vi "HexStringToBoolArray.vi"(0 "Input String":string="FF 55 01", 5 "Fixed Output Size (bytes)":i32=-1, 7 "Reverse Endian?":bool, 11 "Error In":errorcluster) -> (4 "Output Array":bool[][](array[boolean])=[[TRUE, FALSE, FALSE, FALSE, FALSE, FALSE, FALSE, FALSE], [TRUE, FALSE, TRUE, FALSE, TRUE, FALSE, TRUE, FALSE], [TRUE, TRUE, TRUE, TRUE, TRUE, TRUE, TRUE, TRUE]], 15 "Error Out":errorcluster)   [LabVIEW 2016]
panel:
  out "u32 verified":u32=16733441 format="%08x"
  # "Set 'Reverse' if working with hex data where MSB is at end of string."
  # "Pads leading zeroes to output \na larger size, or trims MSB(s) to \noutput a smaller size.\nEx:  For Input \"FF 55 01\": \n       Size 3 yields 0xFF5501\n       Size 2 yields (u16) 0x5501\n       Size 4 yields (u32) 0x00FF5501\n\nDefault (-1) maintains the input size"
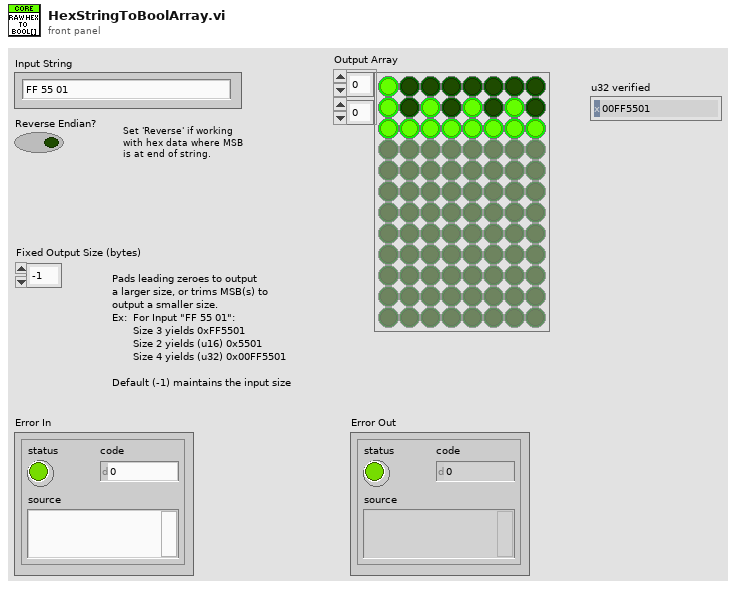
[diagram p1: front panel]
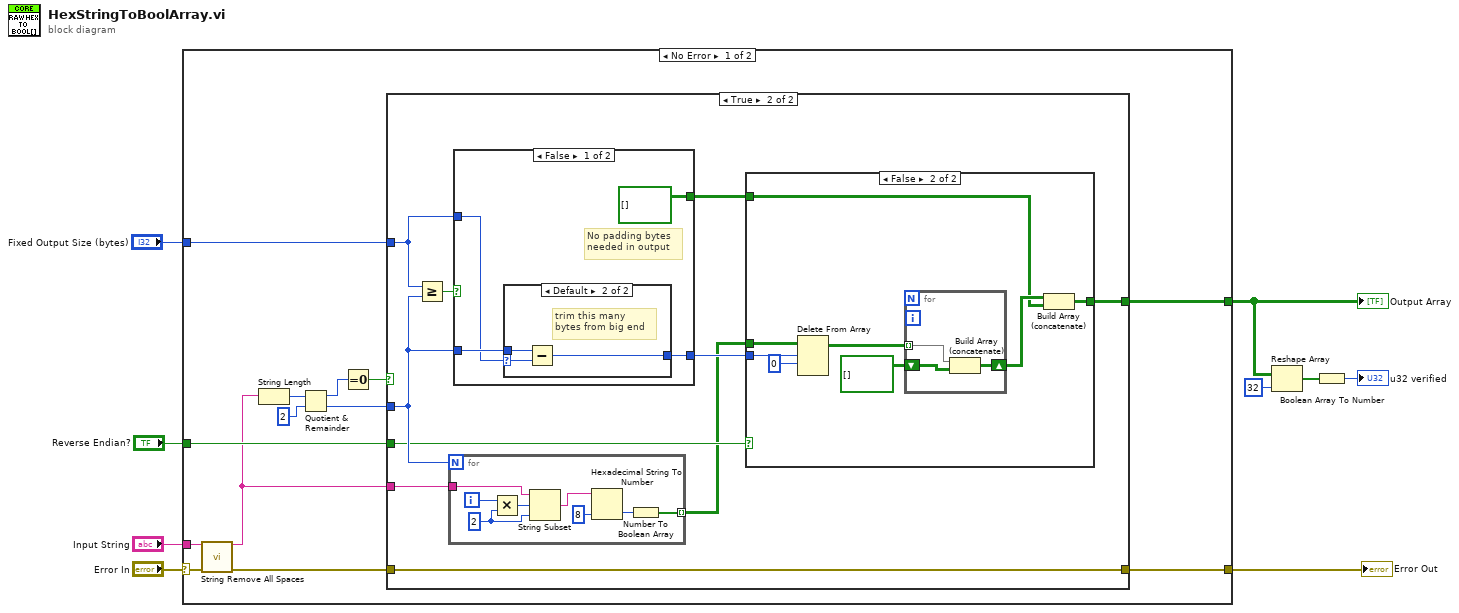
[diagram p0: block diagram]
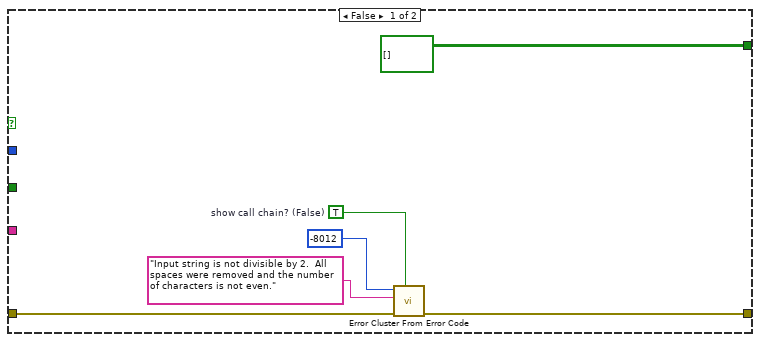
[diagram p2: hidden frame]
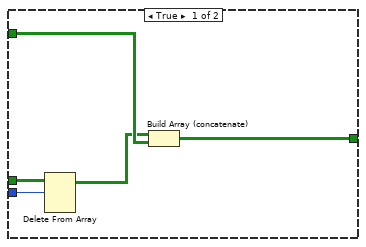
[diagram p3: hidden frame]
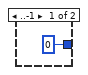
[diagram p4: hidden frame]
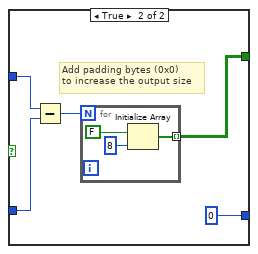
[diagram p5: hidden frame]
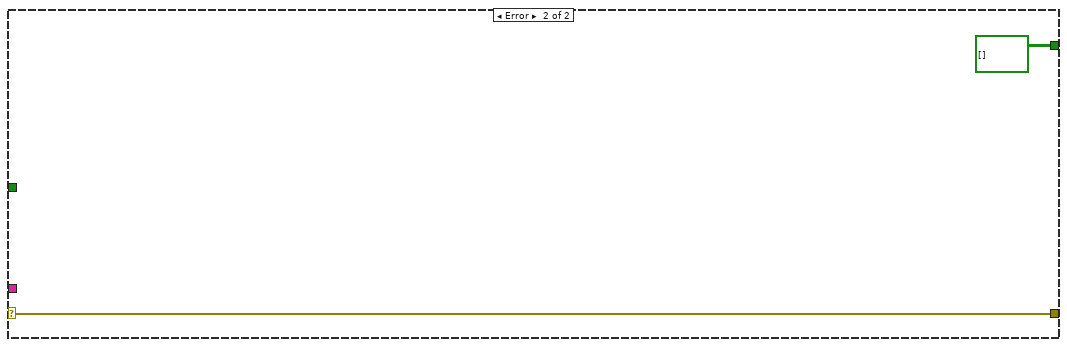
[diagram p6: hidden frame]
diagram:
  n1 = case shown="No Error" "Error In" {
    selector: "Error In" -> [w21 w79]
    tunnel: "Input String" -> [w22 _]
    tunnel: "Fixed Output Size (bytes)" -> [w11 _]
    tunnel: "Reverse Endian?" -> [w14 _]
    tunnel: [w15 bool[][] []] -> w5
    tunnel: [w10 w79] -> w1
    frame No Error {
      n2 = call "String Remove All Spaces.vi"("Input String"=w22, "error in (no error)"=w21) -> ("Spaces Removed"=w13:string, "error out"=w16:errorcluster)  [unwired: 12 in]
      n3 = String Length(string=w13) -> (length=w20:i32)
      n4 = Quotient & Remainder(x=w20, y=2) -> (x-y*floor(x/y)=w18:i32, floor(x/y)=w12:i32)
      n5 = Equal To 0?(x=w18) -> (x = 0?=w17:bool)
      n6 = case shown="True" w17 {
        tunnel: w12 -> [_ w34]
        tunnel: [w28 w38] -> w10
        tunnel: w16 -> [w27 w38]
        tunnel: w14 -> [_ w31]
        tunnel: w13 -> [_ w35]
        tunnel: [bool[][] [] w32] -> w15
        tunnel: w11 -> [_ w37]
        frame False {
          w24 = TRUE  # show call chain? (False)
          n7 = call <vilib>:"Error Cluster From Error Code.vi"("show call chain? (False)"=w24, "error in (no error)"=w27, "error message (\"\")"="Input string is not divisible by 2.  All spaces were removed and the number of characters is not even.", "error code (0)"=-8012) -> ("error out"=w28:errorcluster)  [unwired: 5 in]
        }
        frame True {
          n8 = Greater Or Equal?(x=w37, y=w34) -> (x >= y?=w36:bool)
          n9 = for {
            N: w34 -> [_]
            tunnel: w35 -> [w46]
            tunnel: [w39] -> w29 mode=indexing
            i -> [w43]
            w45 = 2 ("length (rest)")
            n10 = Multiply(x=w43, y=w45) -> (x*y=w44:i32)
            n11 = String Subset(string=w46, offset (0)=w44, length (rest)=w45) -> (substring=w42:string)
            n12 = Hexadecimal String To Number(string=w42, default (0uL)=u8 8 ("default (0 U32)")) -> (number=w40:u8)  [unwired: 1 in, 1 out]
            n13 = Number To Boolean Array(number=w40) -> (Boolean array=w39:bool[])
          }
          n14 = case shown="False" w36 {
            tunnel: w37 -> [w64 w75]
            tunnel: w34 -> [w65 w74]
            tunnel: [bool[][] [] w72] -> w33
            tunnel: [w63 0] -> w30
            frame False {
              # "No padding bytes\nneeded in output"
              n15 = case shown="Default" w64 {
                selector: w64 -> [_ w69]
                tunnel: w65 -> [_ w70]
                tunnel: [0 w68] -> w63
                frame ..-1 {
                }
                frame Default {
                  # "trim this many \nbytes from big end"
                  n16 = Subtract(x=w70, y=w69) -> (x-y=w68:i32)
                }
              }
            }
            frame True {
              # "Add padding bytes (0x0) \nto increase the output size"
              n17 = Subtract(x=w75, y=w74) -> (x-y=w73:i32)
              n18 = for {
                N: w73 -> [_]
                tunnel: [w76] -> w72 mode=indexing
                n19 = Initialize Array(FALSE ("Boolean"), 8 ("x")) -> (w76:bool[])
              }
            }
          }
          n20 = case shown="False" w31 {
            tunnel: w29 -> [w48 w53]
            tunnel: w33 -> [w51 w57]
            tunnel: [w50 w56] -> w32
            tunnel: w30 -> [w49 w54]
            frame True {
              n21 = Delete From Array(array=w48, length=w49) -> (array with subset deleted=w47:bool[][])  [unwired: 2 in, 1 out]
              n22 = Build Array (concatenate)(w47, w51) -> (w50:bool[][])
            }
            frame False {
              n23 = Delete From Array(array=w53, length=w54, index (row)=0) -> (array with subset deleted=w52:bool[][])  [unwired: 1 in, 1 out]
              n24 = for {
                tunnel: w52 -> [w62] mode=indexing
                shift-right: [w60] -> w58
                shift-left: bool[][] [] ("Boolean array") -> [w61]
                n25 = Build Array (concatenate)(w62, w61) -> (w60:bool[][])
              }
              n26 = Build Array (concatenate)(w58, w57) -> (w56:bool[][])
            }
          }
        }
      }
    }
    frame Error {
    }
  }
  "Output Array" <- w5
  "Error Out" <- w1
  n27 = Reshape Array(w5, 32 ("dimension size")) -> (w4:bool[])
  n28 = Boolean Array To Number(Boolean array=w4) -> (number=→"u32 verified":u32)
